vi "Scale Window Trigger 20221110.vi"(10 "scaling coefficients":T1[](array[typedef]), 11 "Sliding Window Trigger":cluster{"Range":dbl, "StartCenter":dbl}[](array[cluster])) -> (3 "Sliding Window Trigger (FXP)":T2[](array[typedef]))   [LabVIEW 2021]
doc: "Scale from double (volts) to digitizer bits"
uses:
  Clusts/ChannelWindowClust.ctl
  <instrlib>/_niInstr/Multirecord Acquisition/Interface/v1/Host/Public/Scaling Coefficient.ctl
  <instrlib>/_niInstr/Multirecord Acquisition/Interface/v1/Host/niInstr Multirecord Acquisition v1 Host.lvclass
panel:
  out "Iteration":i32
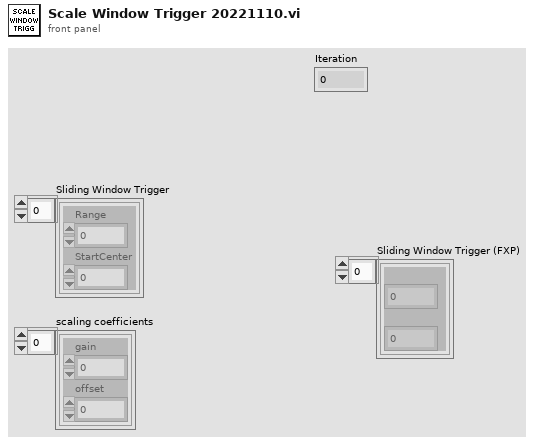
[diagram p1: front panel]
types:
  T1 = typedef "niInstr Multirecord Acquisition v1 Host.lvclass/Scaling Coefficient.ctl" = cluster{"gain":dbl, "offset":dbl}
  T2 = typedef "ChannelWindowClust.ctl" = cluster{"HalfRange":fxp<+/-,18,5>, "StartCenter":fxp<+/-,18,5>}
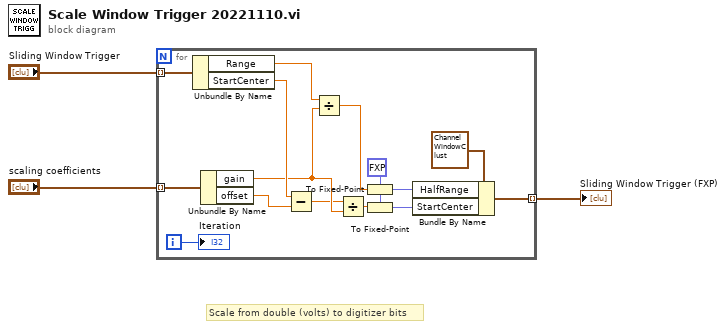
[diagram p0: block diagram]
diagram:
  # "Scale from double (volts) to digitizer bits"
  n1 = for {
    tunnel: "Sliding Window Trigger" -> [w16] mode=indexing
    tunnel: "scaling coefficients" -> [w15] mode=indexing
    tunnel: [w17] -> w3 mode=indexing
    i -> [w4]
    w5 = fxp<+/-,18,5> 0.0 ("fixed-point type")
    n2 = Unbundle By Name(w16) -> ("Range"=w14:dbl, "StartCenter"=w11:dbl)
    n3 = Unbundle By Name(w15) -> ("gain"=w9:dbl, "offset"=w10:dbl)
    n4 = Subtract(x=w11, y=w10) -> (x-y=w8:dbl)
    n5 = Divide(x=w14, y=w9) -> (x/y=w13:dbl)
    n6 = Divide(x=w8, y=w9) -> (x/y=w7:dbl)
    n7 = To Fixed-Point(fixed-point type=w5, number=w13) -> (fixed-point=w12:fxp<+/-,18,5>)
    n8 = To Fixed-Point(fixed-point type=w5, number=w7) -> (fixed-point=w6:fxp<+/-,18,5>)
    n9 = Bundle By Name(cluster=T2 {"HalfRange"=0.0, "StartCenter"=0.0} ("0"), "HalfRange"=w12, "StartCenter"=w6) -> (w17:T2)
    "Iteration" <- w4
  }
  "Sliding Window Trigger (FXP)" <- w3
